vi "Add_Post_Install_Step.vi"(8 "error in (no error)":errorcluster, 11 "IB_RestfulWS in":refnum<class "IB_RestfulWS.lvclass">) -> (0 "error out":errorcluster, 1 "add?":bool, 2 "Pre_Uninstall_Step":refnum<class "IB_Post_Install_Step.lvclass">, 3 "Post_Install_Step":refnum<class "IB_Post_Install_Step.lvclass">)   [LabVIEW 2020, in "IB_RestfulWS.lvclass"]
uses:
  <vilib>/AppBuilder/IB_Classes/Source/Container/Build/RestfulWS/IB_RestfulWS.lvclass
  <vilib>/AppBuilder/IB_Classes/Source/Container/Build/RestfulWS/IB_RestfulWS.lvclass/IB_RestfulWS.ctl
  <vilib>/AppBuilder/IB_Classes/Source/IB_Source.lvclass
  <vilib>/AppBuilder/IB_Classes/Source/Container/IB_Source_Container.lvclass
  e:/builds/penguin/labview/branches/2020/dev/dist/vi.lib/AppBuilder/IB_Classes/Source/Container/Build/IB_Source_Build.lvclass
  e:/builds/penguin/labview/branches/2020/dev/dist/vi.lib/AppBuilder/IB_Classes/Source/Container/IB_Source_Container.lvclass
  e:/builds/penguin/labview/branches/2020/dev/dist/vi.lib/AppBuilder/IB_Classes/Source/IB_Source.lvclass
  e:/builds/penguin/labview/branches/2020/dev/dist/vi.lib/AppBuilder/IB_Classes/Source/Container/Build/RestfulWS/IB_RestfulWS.lvclass
  <vilib>/AppBuilder/IB_Classes/Source/File/CtrFile/IB_CtrFile.lvclass
  e:/builds/penguin/labview/branches/2020/dev/dist/vi.lib/AppBuilder/IB_Classes/Source/File/IB_Source_File.lvclass
  e:/builds/penguin/labview/branches/2020/dev/dist/vi.lib/AppBuilder/IB_Classes/Source/File/CtrFile/IB_CtrFile.lvclass
  <vilib>/AppBuilder/IB_Classes/Post_Install_Step/IB_Post_Install_Step.lvclass
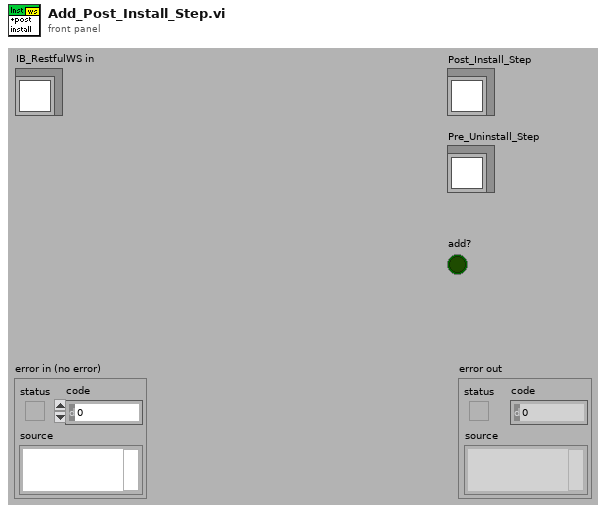
[diagram p1: front panel]
types:
  T1 = typedef "IB_Source_Container.ctl" = cluster{"files":refnum<class "IB_CtrFile.lvclass">[], "previewed?":bool, "preview error?":bool}
  T2 = typedef "IB_Source.ctl" = cluster{"name":string, "sourceTag":string, "destTag":string, "path":path, "eng_installPath":string, "UI_inBuild?":bool, "str ref?":bool}
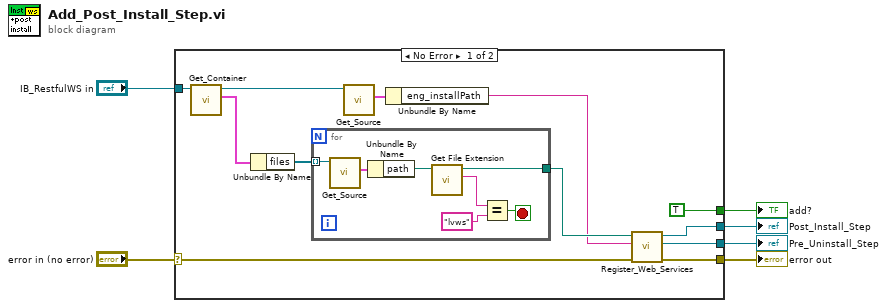
[diagram p0: block diagram]
diagram:
  n1 = case shown="No Error" "error in (no error)" {
    selector: "error in (no error)" -> [w8 w26]
    tunnel: [w7 w26] -> w5
    tunnel: [TRUE ("add?") _] -> w4
    tunnel: "IB_RestfulWS in" -> [w16 _]
    tunnel: [w10 _] -> w2
    tunnel: [w9 _] -> w1
    frame No Error {
      n2 = call <vilib>:"Get_Container.vi"("IB_Source_Container in"=w16) -> ("data"=w14:T1, "IB_Source_Container out"=w15:refnum<class "IB_RestfulWS.lvclass">)  [unwired: 1 in, 8 out]
      n3 = Unbundle By Name(w14) -> ("files"=w13:refnum<class "IB_CtrFile.lvclass">[])
      n4 = for {
        tunnel: w13 -> [w24] mode=indexing
        tunnel: [w19] -> w12
        stop <- w20 stop-if-true
        n5 = call <vilib>:"Get_Source.vi"("IB_Source in"=w24) -> ("data"=w25:T2)  [unwired: 1 in, 9 out]
        n6 = Unbundle By Name(w25) -> ("path"=w23:path)
        n7 = call <vilib>:"Get File Extension.vi"("file"=w23) -> ("lowercase file extension"=w22:string, "dup file"=w19:path)  [unwired: 1 in, 8 out]
        n8 = Equal?(x=w22, y="lvws" ("format string")) -> (x = y?=w20:bool)
      }
      n9 = call <vilib>:"Get_Source.vi"("IB_Source in"=w15) -> ("data"=w17:T2)  [unwired: 1 in, 9 out]
      n10 = Unbundle By Name(w17) -> ("eng_installPath"=w11:string)
      n11 = call <vilib>:"Register_Web_Services.vi"("error in"=w8, "eng_installPath"=w11, "source path"=w12) -> ("error out"=w7:errorcluster, "Pre_Uninstall_Step"=w9:refnum<class "IB_Post_Install_Step.lvclass">, "Post_Install_Step"=w10:refnum<class "IB_Post_Install_Step.lvclass">)  [unwired: 6 in]
    }
    frame Error {
    }
  }
  "error out" <- w5
  "Post_Install_Step" <- w2
  "add?" <- w4
  "Pre_Uninstall_Step" <- w1
